vi "Read Branch Rate - With Two Methods - Returns Total Value.vi"() -> ()   [LabVIEW 2017, in "Cobertura.Tests.lvlib" / "Class.lvlib"]
uses:
  Class.lvlib
  Cobertura/Class/Class.lvclass/Class.ctl
  Cobertura/Class/Read Branch Rate.vi
  <vilib>/PNR/Transparent Assertions/Transparent Assertions/Transparent Assertions.lvlib
  Cobertura/Class/Class.lvclass
  Cobertura/Method/Method.lvclass
panel:
  out "error out":errorcluster
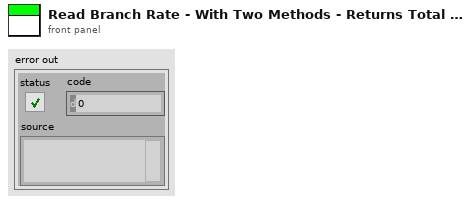
[diagram p1: front panel]
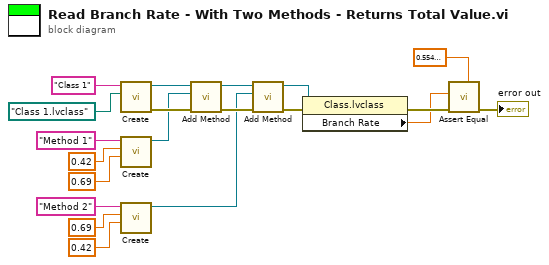
[diagram p0: block diagram]
diagram:
  n1 = call "Create.vi"("Filename"=path "Class 1.lvclass", "Name"="Class 1") -> ("error out"=w19:errorcluster, "Class"=w15:refnum<class "Class.lvclass">)  [unwired: 8 in]
  n2 = call "Create.vi"("Branch Rate"=0.69, "Line Rate"=0.42, "Name"="Method 1") -> ("Method"=w11:refnum<class "Method.lvclass">)  [unwired: 7 in, 1 out]
  n3 = call "Create.vi"("Branch Rate"=0.42, "Line Rate"=0.69, "Name"="Method 2") -> ("Method"=w4:refnum<class "Method.lvclass">)  [unwired: 7 in, 1 out]
  n4 = call "Add Method.vi"("error in (no error)"=w19, "Method"=w11, "Class in"=w15) -> ("error out"=w16:errorcluster, "Class out"=w6:refnum<class "Class.lvclass">)  [unwired: 7 in]
  n5 = call "Add Method.vi"("error in (no error)"=w16, "Method"=w4, "Class in"=w6) -> ("error out"=w7:errorcluster, "Class out"=w5:refnum<class "Class.lvclass">)  [unwired: 7 in]
  n6 = property class="Class.lvclass"(reference=w5, error in=w7) -> (error out=w18:errorcluster, "Branch Rate"=w3:dbl)  [unwired: 1 out]
  n7 = call <vilib>:"Assert Equal.vi"("Expected"=0.5549999999999999 ("Branch Rate"), "error in (no error)"=w18, "Actual"=w3) -> ("error out"=→"error out":errorcluster)  [unwired: 8 in]
